vi "waveformsDObuffer.vi"(1 "DO wf in":digitalwaveform[](array[waveform]), 2 "command":string="clear") -> (0 "DO wf out":digitalwaveform[](array[waveform]))   [LabVIEW 2015]
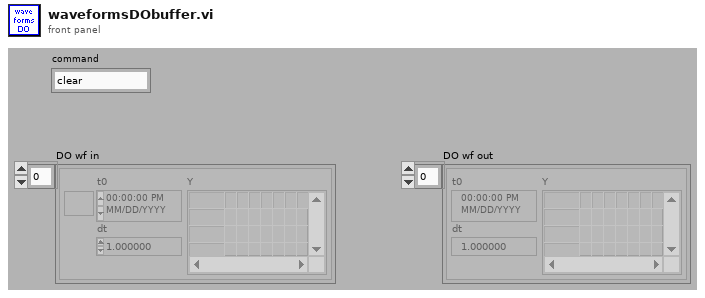
[diagram p1: front panel]
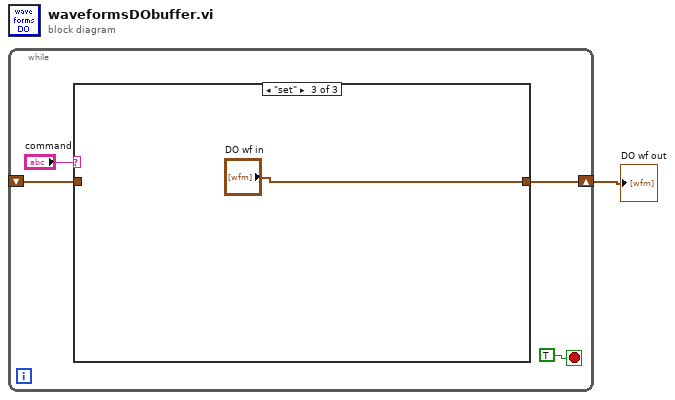
[diagram p0: block diagram]
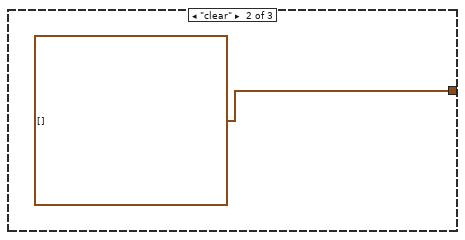
[diagram p3: hidden frame]
diagram:
  n1 = while {
    shift-right: [w3] -> w1
    shift-left: _ -> [w2]
    stop <- TRUE stop-if-true
    n2 = case shown="\"set\"" "command" {
      tunnel: [w6 digitalwaveform[] [] ("Digital waveforms") "DO wf in"] -> w3
      tunnel: w2 -> [w6 _ _]
      frame "get", Default {
      }
      frame "clear" {
      }
      frame "set" {
      }
    }
  }
  "DO wf out" <- w1
